vi "Get Data Variant.vi"(8 "error in (no error)":errorcluster, 11 "Core Transfers Configuration in":refnum<class "Transfer Configuration.lvclass">) -> (0 "error out":errorcluster, 1 "data version":T1, 2 "data":variant, 3 "Core Transfers Configuration out":refnum<class "Transfer Configuration.lvclass">)   [LabVIEW 2019, in "DSF Core.lvlib" / "Transfer Configuration.lvclass"]
uses:
  Transfer Configuration.lvclass
  Typedefs/DSF Version Info.ctl
  Transfer Configuration.lvclass/Transfer Configuration.ctl
  DSF Core.lvlib
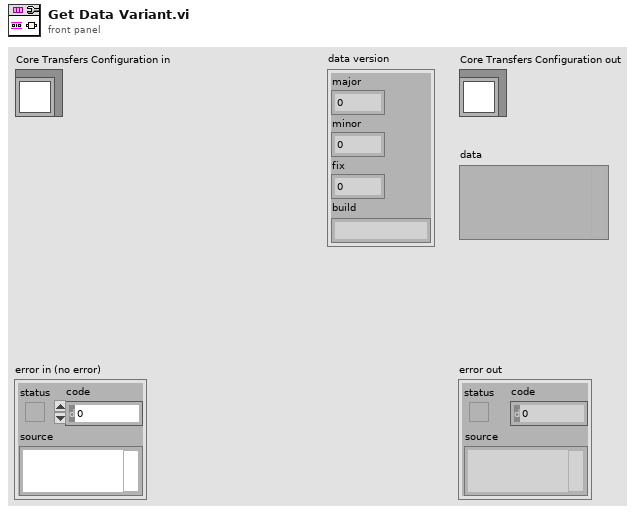
[diagram p1: front panel]
types:
  T1 = typedef "DSF Core.lvlib/DSF Version Info.ctl" = cluster{"major":u32, "minor":u32, "fix":u32, "build":string}
  T2 = typedef "DSF Core.lvlib/Transfer Configuration.lvclass/Core Transfer Configuration.ctl" = cluster{"name":string}
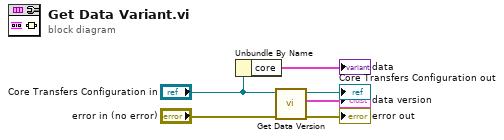
[diagram p0: block diagram]
diagram:
  n1 = Unbundle By Name("Core Transfers Configuration in") -> ("core"=→"data":T2)
  n2 = call-dynamic "Get Data Version.vi"("error in (no error)"="error in (no error)", "Core Transfer Configuration in"="Core Transfers Configuration in") -> ("error out"=→"error out":errorcluster, "data version"=→"data version":T1, "Core Transfer Configuration out"=→"Core Transfers Configuration out":refnum<class "Transfer Configuration.lvclass">)  [unwired: 7 in]
